vi "Read Barcodes.vi"   [LabVIEW 2020, in "feature_detection.lvlib" / "ZXing.lvclass"]
uses:
  ZXing.lvclass
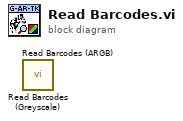
[diagram p0: block diagram]
diagram:
  n1 = call "Read Barcodes (Greyscale).vi"() -> ()  [unwired: 9 in, 3 out]
  n2 = call "Read Barcodes (ARGB).vi"() -> ()  [unwired: 9 in, 3 out]
